vi "ReshapeItemArray.vi"(11 "Array":refnum<class "Link.lvclass">[](array[class])) -> (1 "ring info":refnum<class "RingItem.lvclass">[](array[class]), 3 "item info array":T1(array[cluster]))   [LabVIEW 2009, in "NavScreen.lvlib"]
uses:
  NavScreen.lvlib
  Classes/Link/Link.lvclass
  Classes/ClickableText/ClickableText.lvclass
  Classes/RingItem/RingItem.lvclass
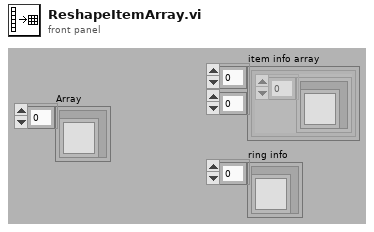
[diagram p1: front panel]
types:
  T1 = cluster{refnum<class "ClickableText.lvclass">[]}[][]
  T2 = typedef "NavScreen.lvlib/PositionCategory.ctl" = enum16{"none", "column 1", "column 2", "ring"}
  T3 = cluster{refnum<class "ClickableText.lvclass">[]}[]
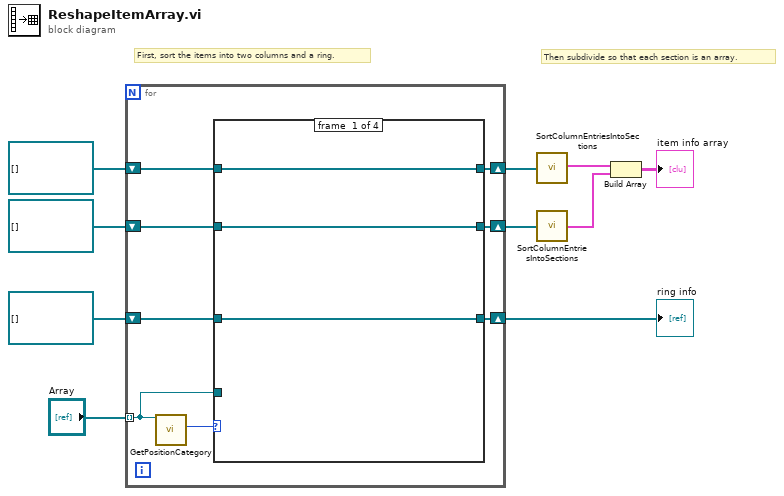
[diagram p0: block diagram]
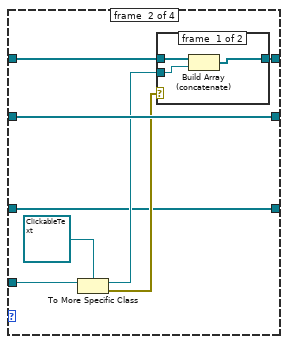
[diagram p2: hidden frame]
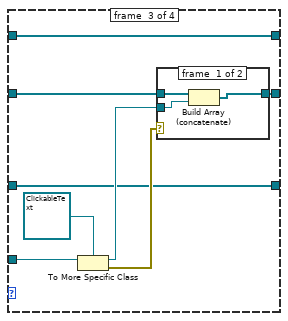
[diagram p4: hidden frame]
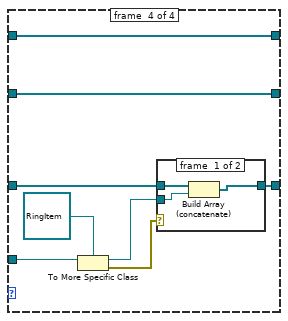
[diagram p6: hidden frame]
diagram:
  # "Then subdivide so that each section is an array."
  # "First, sort the items into two columns and a ring."
  n1 = for {
    tunnel: "Array" -> [w13] mode=indexing
    shift-right: [w16] -> w2
    shift-left: refnum<class "ClickableText.lvclass">[] [] -> [w17]
    shift-right: [w14] -> w1
    shift-left: refnum<class "ClickableText.lvclass">[] [] -> [w15]
    shift-right: [w11] -> w3
    shift-left: refnum<class "RingItem.lvclass">[] [] -> [w12]
    n2 = call-dynamic "GetPositionCategory.vi"("Link in"=w13) -> ("position"=w18:T2)  [unwired: 8 in, 2 out]
    n3 = case shown="\"none\"" w18 {
      tunnel: w17 -> [w21 w29 w36 w49]
      tunnel: w13 -> [_ w26 w41 w53]
      tunnel: [w21 w28 w36 w49] -> w16
      tunnel: w15 -> [w20 w27 w37 w48]
      tunnel: [w20 w27 w35 w48] -> w14
      tunnel: w12 -> [w19 w22 w34 w47]
      tunnel: [w19 w22 w34 w46] -> w11
      frame #0 {
      }
      frame #1 {
        n4 = To More Specific Class(target class=refnum<class "ClickableText.lvclass"> refnum ("GettingStartedWindow.lvlib:ClickableText.lvclass"), reference=w26) -> (specific class reference=w24:refnum<class "ClickableText.lvclass">, error out=w23:errorcluster)  [unwired: 1 in]
        n5 = case shown="No Error" w23 {
          tunnel: w29 -> [w32 w33]
          tunnel: [w31 w33] -> w28
          tunnel: w24 -> [w30 _]
          frame #0 {
            n6 = Build Array (concatenate)(w32, w30) -> (w31:refnum<class "ClickableText.lvclass">[])
          }
          frame #1 {
          }
        }
      }
      frame #2 {
        n7 = To More Specific Class(target class=refnum<class "ClickableText.lvclass"> refnum ("GettingStartedWindow.lvlib:ClickableText.lvclass"), reference=w41) -> (specific class reference=w39:refnum<class "ClickableText.lvclass">, error out=w38:errorcluster)  [unwired: 1 in]
        n8 = case shown="No Error" w38 {
          tunnel: w37 -> [w44 w45]
          tunnel: [w43 w45] -> w35
          tunnel: w39 -> [w42 _]
          frame #0 {
            n9 = Build Array (concatenate)(w44, w42) -> (w43:refnum<class "ClickableText.lvclass">[])
          }
          frame #1 {
          }
        }
      }
      frame #3 {
        n10 = To More Specific Class(target class=refnum<class "RingItem.lvclass"> refnum ("GettingStartedWindow.lvlib:RingItem.lvclass"), reference=w53) -> (specific class reference=w51:refnum<class "RingItem.lvclass">, error out=w50:errorcluster)  [unwired: 1 in]
        n11 = case shown="No Error" w50 {
          tunnel: w47 -> [w56 w57]
          tunnel: [w55 w57] -> w46
          tunnel: w51 -> [w54 _]
          frame #0 {
            n12 = Build Array (concatenate)(w56, w54) -> (w55:refnum<class "RingItem.lvclass">[])
          }
          frame #1 {
          }
        }
      }
    }
  }
  "ring info" <- w3
  n13 = call "SortColumnEntriesIntoSections.vi"("Array"=w2) -> ("Sorted Array"=w6:T3)
  n14 = call "SortColumnEntriesIntoSections.vi"("Array"=w1) -> ("Sorted Array"=w4:T3)
  n15 = Build Array(w6, w4) -> (→"item info array":T1)
